vi "Import - Tx Packet.vi"(7 "Tx Packet":T1 {"threadOptions"."pclDecimation" max=16 step=1; "threadOptions"."loopPeriod" max=16 step=1; "threadOptions"."targetPriority" min=-2 max=16 step=1; "threadOptions"."targetProcessor" min=-2 max=16 step=1; "Endianness" items=["big-endian"=0, "little-endian"=2]}, 8 "error in (no error)":errorcluster, 11 "Device Item Ref in":T13 format="%.0x") -> (0 "error out":errorcluster)   [LabVIEW 2019, in "UDP-Custom-Device System Explorer.lvlib"]
uses:
  UDP-Custom-Device System Explorer.lvlib
  <vilib>/NI VeriStand/Custom Device API/Custom Device Item Ref.ctl
  Types/XML - New/ImpExp - Tx Packet Data.ctl
  <vilib>/NI VeriStand/Custom Device API/Custom Device Item Info.ctl
  Shared/Types/Shared - Channel Data Type.ctl
  Shared/Types/Shared - Buffered.PacketInfo.ctl
  Shared/Types/Shared - Pointer Encoding.ctl
  Shared/Types/Shared - Receive Buffer Options.ctl
  Shared/Types/Shared - Transmit Buffer Options.ctl
  Shared/Types/Shared - Transmit Flag Options.ctl
  Shared/Types/Shared - Transmit Echo Options.ctl
  Types/Threading/Thread Configuration.ctl
  Types/Threading/Thread Sync Reference.ctl
  Shared/Types/Shared - Thread Management.ctl
  Property Accessors/Shared Packet Accessors.lvlib
  Property Accessors/Tx Packet Accessors.lvlib
  <vilib>/NI VeriStand/Custom Device API/Custom Device API.lvlib
  <vilib>/NI VeriStand/Custom Device Tools/Custom Device Utility Library/Custom Device Utility Library.lvlib
  Shared/UDP-Custom-Device Shared.lvlib
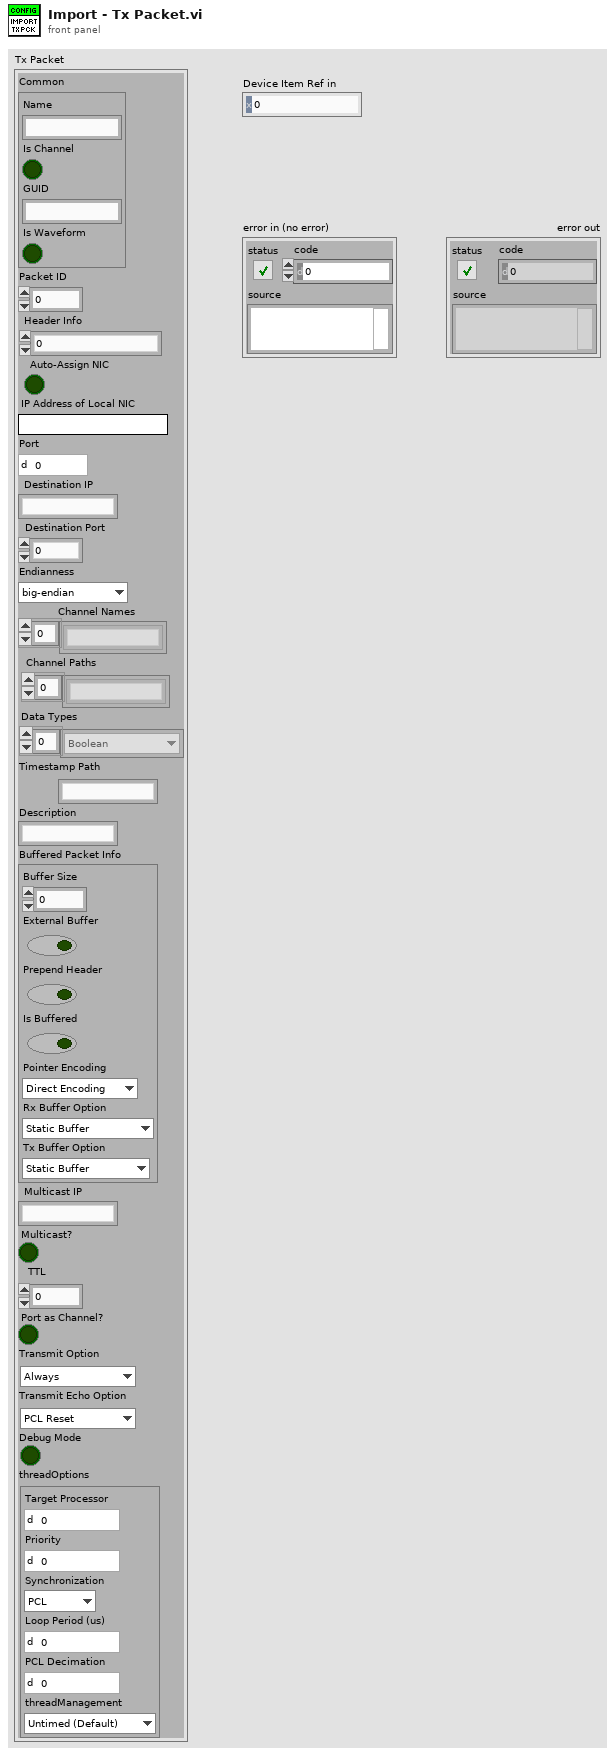
[diagram p1: front panel]
types:
  T1 = typedef "UDP-Custom-Device System Explorer.lvlib/ImpExp - Tx Packet Data.ctl" = cluster{"Common":T2, "Packet ID":i32, "Header Info":u32, "Auto-Assign NIC":bool, "IP Address of Local NIC":string, "Port":u16, "Destination IP":string, "Destination Port":u16, "Endianness":u16, "Channel Names":string[], "Channel Paths":string[], "Data Types":T3[], "Timestamp Path":string, "Description":string, "Buffered Packet Info":T4, "Multicast IP":string, "Multicast?":bool, "TTL":u16, "Port as Channel?":bool, "Transmit Option":T8, "Transmit Echo Option":T9, "Debug Mode":bool, "threadOptions":T10}
  T2 = typedef "Custom Device API.lvlib/Custom Device Item Info.ctl" = cluster{"Name":string, "Is Channel":bool, "GUID":string, "Is Waveform":bool}
  T3 = typedef "UDP-Custom-Device Shared.lvlib/Shared - Channel Data Type.ctl" = enum16{"Boolean", "Single", "Double", "I8", "I16", "I32", "I64", "U8", "U16", "U32", "U64"}
  T4 = typedef "UDP-Custom-Device Shared.lvlib/Shared - Buffered.PacketInfo.ctl" = cluster{"Buffer Size":i32, "External Buffer":bool, "Prepend Header":bool, "Is Buffered":bool, "Pointer Encoding":T5, "Rx Buffer Option":T6, "Tx Buffer Option":T7}
  T5 = typedef "UDP-Custom-Device Shared.lvlib/Shared - Pointer Encoding.ctl" = enum16{"Direct Encoding", "Conversion Encoding"}
  T6 = typedef "UDP-Custom-Device Shared.lvlib/Shared - Receive Buffer Options.ctl" = enum16{"Static Buffer", "Circular Buffer", "Circular Buffer + Size", "Internal Cache", "Internal Cache + Size", "Ping Pong", "Ping Pong + Size"}
  T7 = typedef "UDP-Custom-Device Shared.lvlib/Shared - Transmit Buffer Options.ctl" = enum16{"Static Buffer", "FIFO Buffer", "FIFO Buffer + Port"}
  T8 = typedef "UDP-Custom-Device Shared.lvlib/Shared - Transmit Flag Options.ctl" = enum16{"Always", "One-Shot", "Toggle"}
  T9 = typedef "UDP-Custom-Device Shared.lvlib/Shared - Transmit Echo Options.ctl" = enum16{"PCL Reset", "Counter", "Mirror"}
  T10 = typedef "UDP-Custom-Device System Explorer.lvlib/Thread Configuration.ctl" = cluster{"targetProcessor":i8, "targetPriority":i16, "Synchronization":T11, "loopPeriod":u32, "pclDecimation":u16, "threadManagement":T12}
  T11 = typedef "UDP-Custom-Device System Explorer.lvlib/Thread Sync Reference.ctl" = enum16{"PCL", "Async"}
  T12 = typedef "UDP-Custom-Device Shared.lvlib/Shared - Thread Management.ctl" = enum16{"Untimed (Default)", "Timed (High Priority)"}
  T13 = typedef "Custom Device API.lvlib/Custom Device Item Ref.ctl" = u64
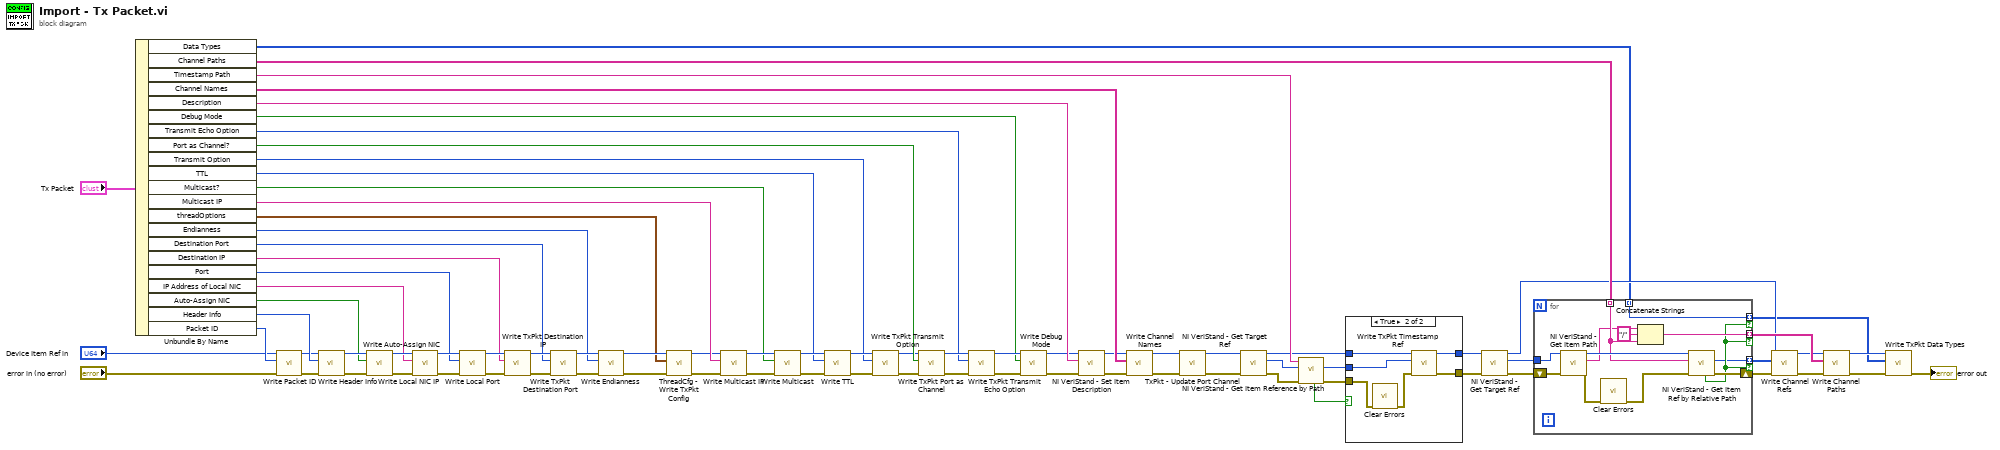
[diagram p0: block diagram]
diagram:
  n1 = Unbundle By Name("Tx Packet") -> ("Data Types"=w35:T3[], "Channel Paths"=w43:string[], "Timestamp Path"=w50:string, "Channel Names"=w56:string[], "Description"=w59:string, "Debug Mode"=w6:bool, "Transmit Echo Option"=w11:T9, "Port as Channel?"=w23:bool, "Transmit Option"=w18:T8, "TTL"=w24:u16, "Multicast?"=w25:bool, "Multicast IP"=w26:string, "threadOptions"=w1:T10, "Endianness"=w60:u16, "Destination Port"=w63:u16, "Destination IP"=w64:string, "Port"=w65:u16, "IP Address of Local NIC"=w66:string, "Auto-Assign NIC"=w75:bool, "Header Info"=w80:u32, "Packet ID"=w81:i32)
  n2 = call "Write Packet ID.vi"("error in (no error)"="error in (no error)", "Packet ID"=w81, "Node Ptr"="Device Item Ref in") -> ("error out"=w78:errorcluster, "Node Ptr out"=w79:T13)  [unwired: 7 in]
  n3 = call "Write Header Info.vi"("error in (no error)"=w78, "Header Info"=w80, "Node Ptr"=w79) -> ("error out"=w76:errorcluster, "Node Ptr out"=w77:T13)  [unwired: 7 in]
  n4 = call "Write Auto-Assign NIC.vi"("error in (no error)"=w76, "Auto-Assign NIC"=w75, "Node Ptr"=w77) -> ("error out"=w70:errorcluster, "Node Ptr out"=w74:T13)  [unwired: 7 in]
  n5 = call "Write Local NIC IP.vi"("error in (no error)"=w70, "IP Address of Local NIC"=w66, "Node Ptr"=w74) -> ("error out"=w69:errorcluster, "Node Ptr out"=w73:T13)  [unwired: 7 in]
  n6 = call "Write Local Port.vi"("error in (no error)"=w69, "Port"=w65, "Node Ptr"=w73) -> ("error out"=w68:errorcluster, "Node Ptr out"=w72:T13)  [unwired: 7 in]
  n7 = call "Write TxPkt Destination IP.vi"("error in (no error)"=w68, "Destination IP"=w64, "Node Ptr"=w72) -> ("error out"=w67:errorcluster, "Node Ptr out"=w71:T13)  [unwired: 7 in]
  n8 = call "Write TxPkt Destination Port.vi"("error in (no error)"=w67, "Destination Port"=w63, "Node Ptr"=w71) -> ("error out"=w61:errorcluster, "Node Ptr out"=w62:T13)  [unwired: 7 in]
  n9 = call "Write Endianness.vi"("error in (no error)"=w61, "Endianness"=w60, "Node Ptr"=w62) -> ("error out"=w4:errorcluster, "Node Ptr out"=w5:T13)  [unwired: 7 in]
  n10 = call "ThreadCfg - Write TxPkt Config.vi"("error in (no error)"=w4, "threadOptions"=w1, "Node Ptr In"=w5) -> ("error out"=w2:errorcluster, "Node Ptr Out"=w3:T13)  [unwired: 7 in]
  n11 = call "Write Multicast IP.vi"("error in (no error)"=w2, "Multicast IP Address"=w26, "Node Ptr"=w3) -> ("error out"=w30:errorcluster, "Node Ptr out"=w28:T13)  [unwired: 7 in]
  n12 = call "Write Multicast.vi"("error in (no error)"=w30, "Multicast"=w25, "Node Ptr"=w28) -> ("error out"=w29:errorcluster, "Node Ptr out"=w27:T13)  [unwired: 7 in]
  n13 = call "Write TTL.vi"("error in (no error)"=w29, "TTL"=w24, "Node Ptr"=w27) -> ("error out"=w22:errorcluster, "Node Ptr out"=w20:T13)  [unwired: 7 in]
  n14 = call "Write TxPkt Transmit Option.vi"("error in (no error)"=w22, "Transmit Options"=w18, "Node Ptr"=w20) -> ("error out"=w21:errorcluster, "Node Ptr out"=w19:T13)  [unwired: 7 in]
  n15 = call "Write TxPkt Port as Channel.vi"("error in (no error)"=w21, "Port as Channel"=w23, "Node Ptr"=w19) -> ("error out"=w12:errorcluster, "Node Ptr out"=w13:T13)  [unwired: 7 in]
  n16 = call "Write TxPkt Transmit Echo Option.vi"("error in (no error)"=w12, "Transmit Echo Options"=w11, "Node Ptr"=w13) -> ("error out"=w8:errorcluster, "Node Ptr out"=w10:T13)  [unwired: 7 in]
  n17 = call "Write Debug Mode.vi"("error in (no error)"=w8, "Debug Mode"=w6, "Node Ptr"=w10) -> ("error out"=w7:errorcluster, "Node Ptr out"=w9:T13)  [unwired: 7 in]
  n18 = call <vilib>:"NI VeriStand - Set Item Description.vi"("error in (no error)"=w7, "Description"=w59, "Item Ref in"=w9) -> ("error out"=w54:errorcluster, "Item Ref out"=w55:T13)  [unwired: 6 in, 1 out]
  n19 = call "Write Channel Names.vi"("error in (no error)"=w54, "Channel Names"=w56, "Node Ptr"=w55) -> ("error out"=w15:errorcluster, "Node Ptr out"=w17:T13)  [unwired: 7 in]
  n20 = call "TxPkt - Update Port Channel.vi"("error in (no error)"=w15, "Packet Ref in"=w17) -> ("error out"=w14:errorcluster, "Packet Ref out"=w16:T13)  [unwired: 8 in]
  n21 = call <vilib>:"NI VeriStand - Get Target Ref.vi"("error in"=w14, "Item Ref in"=w16) -> ("error out"=w52:errorcluster, "Target Ref"=w53:T13, "Item Ref out"=w49:T13)  [unwired: 6 in, 1 out]
  n22 = call <vilib>:"NI VeriStand - Get Item Reference by Path.vi"("error in (no error)"=w52, "Root Ref"=w53, "Item Path in"=w50) -> ("error out"=w51:errorcluster, "Item Ref"=w48:T13, "Found"=w41:bool)  [unwired: 5 in, 1 out]
  n23 = case shown="True" w41 {
    tunnel: w51 -> [w83 w90]
    tunnel: w49 -> [w84 w89]
    tunnel: w48 -> [_ w88]
    tunnel: [w84 w86] -> w47
    tunnel: [w83 w85] -> w46
    frame False {
    }
    frame True {
      n24 = call <vilib>:"Clear Errors.vi"("error in (no error)"=w90) -> ("error out"=w87:errorcluster)  [unwired: 5 in, 1 out]
      n25 = call "Write TxPkt Timestamp Ref.vi"("error in (no error)"=w87, "Dependent Node Ref"=w88, "Node Ptr"=w89) -> ("error out"=w85:errorcluster, "Node Ptr out"=w86:T13)  [unwired: 7 in]
    }
  }
  n26 = call <vilib>:"NI VeriStand - Get Target Ref.vi"("error in"=w46, "Item Ref in"=w47) -> ("error out"=w44:errorcluster, "Target Ref"=w45:T13, "Item Ref out"=w39:T13)  [unwired: 6 in, 1 out]
  n27 = for {
    tunnel: w45 -> [w103]
    tunnel: w43 -> [w93] mode=indexing
    tunnel: [w99] -> w42 mode=indexing if=w95
    tunnel: [w94] -> w40 mode=indexing if=w95
    shift-right: [w96] -> w36
    shift-left: w44 -> [w102]
    tunnel: w35 -> [w100] mode=indexing
    tunnel: [w100] -> w31 mode=indexing if=w95
    n28 = call <vilib>:"NI VeriStand - Get Item Path.vi"("error in (no error)"=w102, "Item Ref in"=w103) -> ("error out"=w101:errorcluster, "Path"=w92:string, "Item Ref out"=w98:T13)  [unwired: 6 in, 1 out]
    n29 = call <vilib>:"Clear Errors.vi"("error in (no error)"=w101) -> ("error out"=w97:errorcluster)  [unwired: 5 in, 1 out]
    n30 = Concatenate Strings(w92, "/" ("string"), w93) -> (w99:string)
    n31 = call <vilib>:"NI VeriStand - Get Item Ref by Relative Path.vi"("error in"=w97, "Relative Item Path"=w93, "Section Ref in"=w98) -> ("error out"=w96:errorcluster, "Item Ref"=w94:T13, "Found"=w95:bool)  [unwired: 5 in, 1 out]
  }
  n32 = call "Write Channel Refs.vi"("error in (no error)"=w36, "Dependent Node Refs"=w40, "Node Ptr"=w39) -> ("error out"=w37:errorcluster, "Node Ptr out"=w38:T13)  [unwired: 7 in]
  n33 = call "Write Channel Paths.vi"("error in (no error)"=w37, "Channel Paths"=w42, "Node Ptr"=w38) -> ("error out"=w34:errorcluster, "Node Ptr out"=w32:T13)  [unwired: 7 in]
  n34 = call "Write TxPkt Data Types.vi"("error in (no error)"=w34, "Data Types"=w31, "Node Ptr"=w32) -> ("error out"=→"error out":errorcluster)  [unwired: 7 in, 1 out]
